vi "MSEncoder Case-24-CLFreqScan.vi"(8 "error in (no error)":errorcluster, 9 "ParamValIn":variant, 11 "MSEncoder in":refnum<class "MSEncoder.lvclass">) -> (0 "error out":errorcluster, 3 "MSEncoder out":refnum<class "MSEncoder.lvclass">)   [LabVIEW 2018, in "MSEncoder.lvclass"]
uses:
  MSEncoder.lvclass
  Ctl/MSEditorParam CLFreqScan.ctl
  PublicSubVI/Ctl/MathieuEqParam.ctl
  MSEncoder.lvclass/MSEncoder.ctl
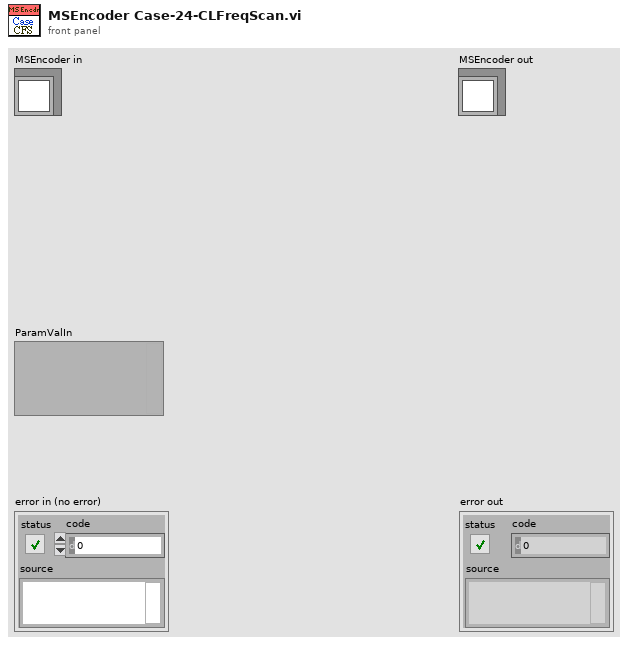
[diagram p1: front panel]
types:
  T1 = typedef "MSEditorParam CLFreqScan.ctl" = cluster{"targetfreq":ext, "time":ext}
  T2 = typedef "MathieuEqParam.ctl" = cluster{"mz(Th)":ext, "Amp(V)":ext, "Freq(Hz)":ext, "Beta":ext, "r_0 (mm)":ext, "z_0 (mm)":ext}
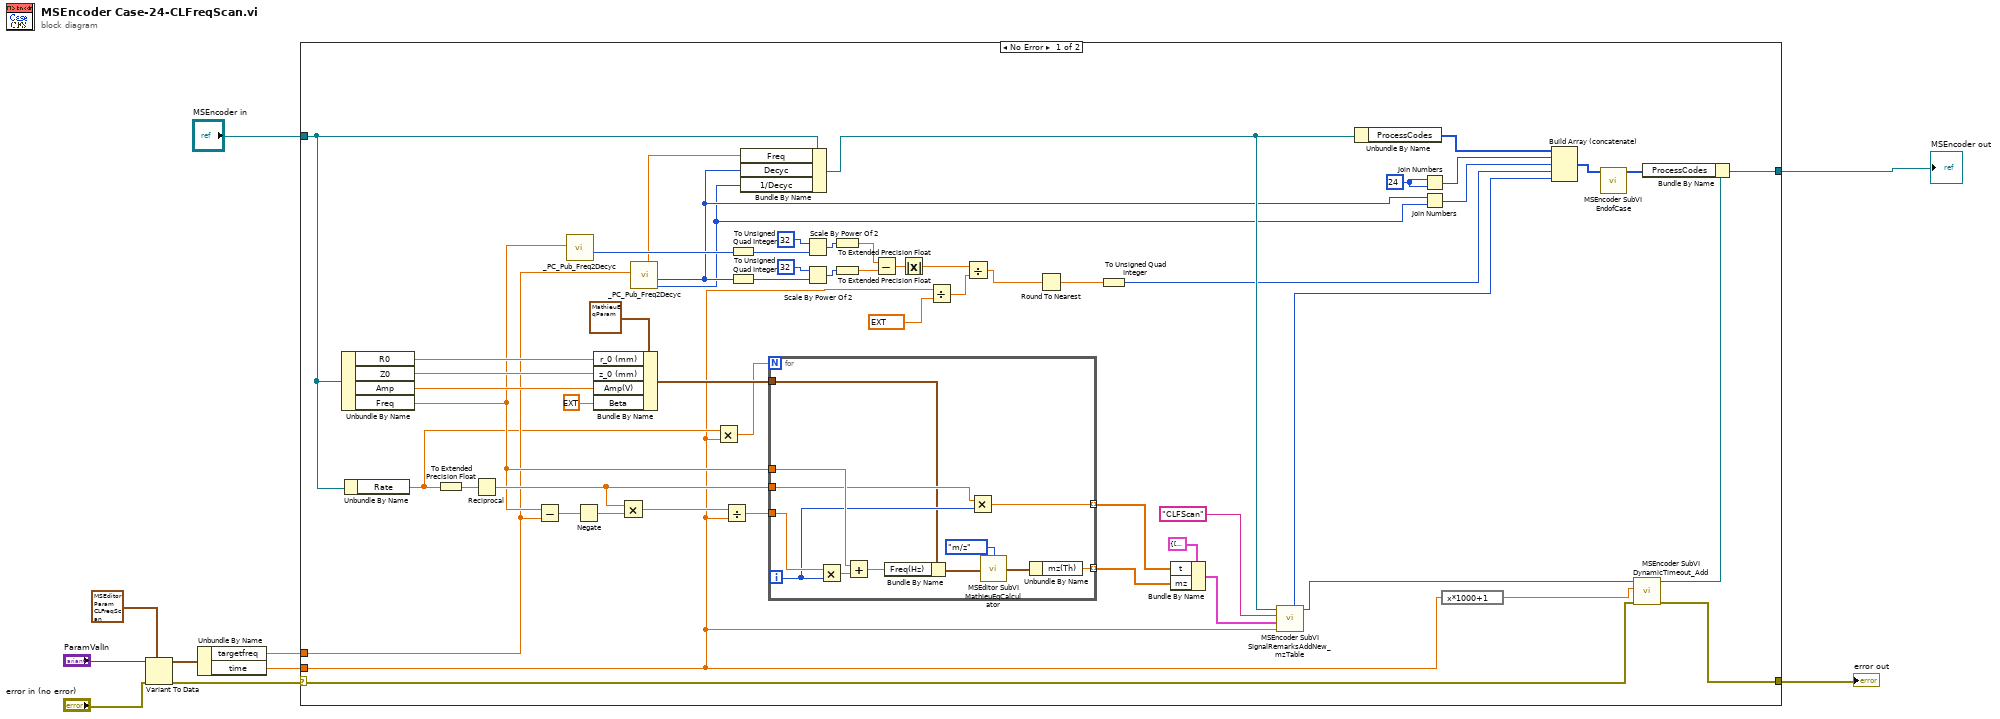
[diagram p0: block diagram]
diagram:
  n1 = Variant To Data(error in="error in (no error)", type=T1 {"targetfreq"=0.0, "time"=1.0} ("ParamValueType"), Variant="ParamValIn") -> (data=w4:T1, error out=w3:errorcluster)
  n2 = Unbundle By Name(w4) -> ("targetfreq"=w1:ext, "time"=w9:ext)
  n3 = case shown="No Error" w3 {
    selector: w3 -> [w53 w80]
    tunnel: "MSEncoder in" -> [w28 w79]
    tunnel: [w54 w80] -> w10
    tunnel: [w66 w79] -> w7
    tunnel: w9 -> [w18 _]
    tunnel: w1 -> [w26 _]
    frame No Error {
      w58 = u32 24
      n4 = Unbundle By Name(w28) -> ("R0"=w65:ext, "Z0"=w64:ext, "Amp"=w63:ext, "Freq"=w40:ext)
      n5 = Unbundle By Name(w28) -> ("Rate"=w19:dbl)
      n6 = To Extended Precision Float(1:w19) -> (0:w47:ext)
      n7 = Reciprocal(x=w47) -> (1/x=w46:ext)
      n8 = Subtract(x=w40, y=w26) -> (x-y=w50:ext)
      n9 = call "_PC_Pub_Freq2Decyc.vi"("Freq"=w40) -> ("Decyc*2^32"=w39:u32)  [unwired: 4 in, 4 out]
      n10 = Negate(x=w50) -> (-x=w49:ext)
      n11 = Bundle By Name(cluster=T2 {"mz(Th)"=0.0, "Amp(V)"=330.0, "Freq(Hz)"=0.0, "Beta"=1.0, "r_0 (mm)"=10.0, "z_0 (mm)"=7.0710678118654755} ("Parametres in"), "r_0 (mm)"=w65, "z_0 (mm)"=w64, "Amp(V)"=w63, "Beta"=ext 1.0) -> (w51:T2)
      n12 = Multiply(x=w46, y=w49) -> (x*y=w48:ext)
      n13 = call "_PC_Pub_Freq2Decyc.vi"("Freq"=w26) -> ("(1/Decyc)*2^8"=w11:u32, "Decyc*2^32"=w12:u32, "Actual Freq"=w25:dbl)  [unwired: 4 in, 2 out]
      n14 = Multiply(x=w19, y=w18) -> (x*y=w17:ext)
      n15 = Divide(x=w48, y=w18) -> (x/y=w45:ext)
      n16 = To Unsigned Quad Integer(1:w39) -> (0:w35:u64)
      n17 = To Unsigned Quad Integer(1:w12) -> (0:w37:u64)
      n18 = Bundle By Name(cluster=w28, "Freq"=w25, "Decyc"=w12, "1/Decyc"=w11) -> (w27:refnum<class "MSEncoder.lvclass">)
      n19 = for {
        N: w17 -> [_]
        tunnel: w51 -> [w67]
        tunnel: w46 -> [w72]
        tunnel: w45 -> [w78]
        tunnel: w40 -> [w76]
        tunnel: [w70] -> w41 mode=indexing
        tunnel: [w69] -> w42 mode=indexing
        i -> [w71]
        n20 = Multiply(x=w78, y=w71) -> (x*y=w77:ext)
        n21 = Add(x=w76, y=w77) -> (x+y=w74:ext)
        n22 = Bundle By Name(cluster=w67, "Freq(Hz)"=w74) -> (w73:T2)
        n23 = Multiply(x=w72, y=w71) -> (x*y=w70:ext)
        n24 = call "MSEditor SubVI MathieuEqCalculator.vi"("Target (Freq)"=enum16{"m/z", "Volt", "Freq", "Beta"}."m/z", "Parametres in"=w73) -> ("Parametres out"=w75:T2)  [unwired: 2 in]
        n25 = Unbundle By Name(w75) -> ("mz(Th)"=w69:ext)
      }
      n26 = Scale By Power Of 2(n=i16 32, x=w35) -> (x*2^n=w34:u64)
      n27 = Scale By Power Of 2(n=i16 32, x=w37) -> (x*2^n=w33:u64)
      n28 = To Extended Precision Float(1:w34) -> (0:w31:ext)
      n29 = To Extended Precision Float(1:w33) -> (0:w32:ext)
      n30 = Subtract(x=w31, y=w32) -> (x-y=w30:ext)
      n31 = Absolute Value(x=w30) -> (abs(x)=w14:ext)
      n32 = Divide(x=w18, y=ext 2.5e-8 ("x")) -> (x/y=w15:ext)
      n33 = Divide(x=w14, y=w15) -> (x/y=w13:ext)
      n34 = Round To Nearest(number=w13) -> (nearest integer value=w29:ext)
      n35 = To Unsigned Quad Integer(1:w29) -> (0:w23:u64)
      n36 = Bundle By Name(cluster=cluster{"t":dbl[], "mz":dbl[], "beta":dbl[]} {"t"=[], "mz"=[], "beta"=[]} ("mzTable"), "t"=w41, "mz"=w42) -> (w43:cluster{"t":dbl[], "mz":dbl[], "beta":dbl[]})
      n37 = call "MSEncoder SubVI SignalRemarksAddNew_mzTable.vi"("Scan time"=w18, "mzTable"=w43, "Label"="CLFScan", "MSEncoder in"=w27) -> ("MSEncoder out"=w20:refnum<class "MSEncoder.lvclass">, "Len"=w22:u32)  [unwired: 6 in]
      n38 = Unbundle By Name(w27) -> ("ProcessCodes"=w57:u64[])
      n39 = Join Numbers(hi=w58, lo=w58) -> ((hi.lo)=w61:u64)
      n40 = Join Numbers(hi=w12, lo=w11) -> ((hi.lo)=w24:u64)
      n41 = expression code="x*1000+1"(w18) -> (w55:ext)
      n42 = Build Array (concatenate)(w57, w61, w24, w23, w22) -> (w60:u64[])
      n43 = call "MSEncoder SubVI EndofCase.vi"("Case codes"=w60) -> ("Case codes with end"=w59:u64[])  [unwired: 9 in, 1 out]
      n44 = call "MSEncoder SubVI DynamicTimeout_Add.vi"("error in (no error)"=w53, "Timeout_ms"=w55, "MSEncoder"=w20) -> ("error out"=w54:errorcluster, "MSEncoder"=w56:refnum<class "MSEncoder.lvclass">)  [unwired: 7 in]
      n45 = Bundle By Name(cluster=w56, "ProcessCodes"=w59) -> (w66:refnum<class "MSEncoder.lvclass">)
    }
    frame Error {
    }
  }
  "error out" <- w10
  "MSEncoder out" <- w7
